vi "HelloWorldJP.vi"() -> ()   [LabVIEW 2015]
panel:
  out "?":string
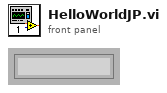
[diagram p1: front panel]
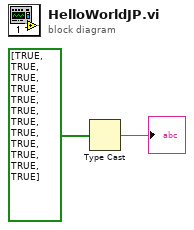
[diagram p0: block diagram]
diagram:
  n1 = Type Cast(x=bool[] [TRUE, TRUE, TRUE, TRUE, TRUE, TRUE, TRUE, TRUE, TRUE, TRUE, TRUE, TRUE] ("*(type *) &x")) -> (*(type *) &x=→"?":string)  [unwired: 1 in]
